vi "ConvertImageToJpg.vi"(11 "buffer":string) -> (1 "image data":T1, 3 "new picture":picture)   [LabVIEW 2017]
uses:
  <vilib>/picture/picture.llb/imagedata.ctl
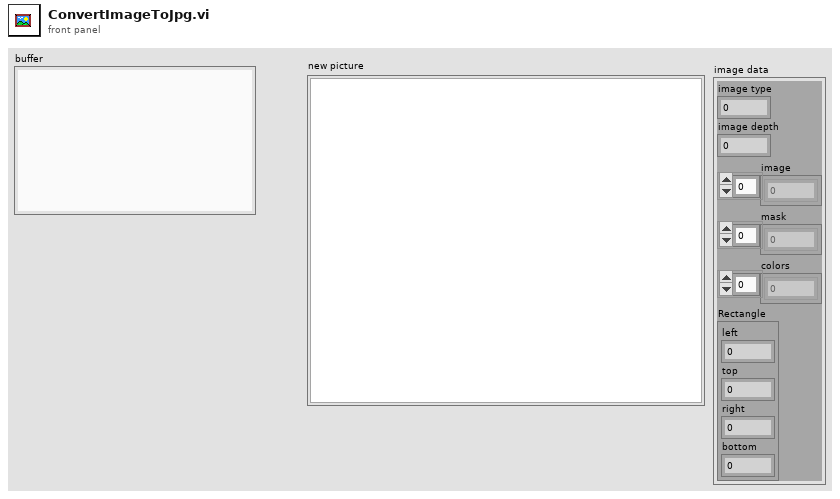
[diagram p1: front panel]
types:
  T1 = typedef "imagedata.ctl" = cluster{"image type":i32, "image depth":i32, "image":u8[], "mask":u8[], "colors":u32[], "Rectangle":cluster{"left":i16, "top":i16, "right":i16, "bottom":i16}}
  T2 = enum16{"big-endian, network order", "native, host order", "little-endian"}
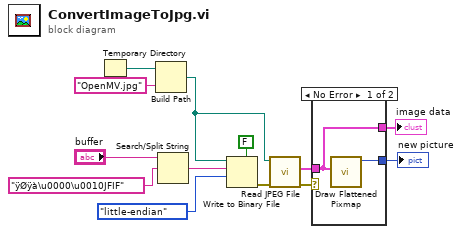
[diagram p0: block diagram]
diagram:
  n1 = Temporary Directory() -> (w4:path)
  n2 = Build Path(base path=w4, name or relative path="OpenMV.jpg") -> (appended path=w2:path)
  n3 = Search/Split String(string="buffer", search string/char (-)="ÿØÿà\u0000\u0010JFIF") -> (match + rest of string=w6:string)  [unwired: 1 in, 2 out]
  n4 = Write to Binary File(file (use dialog)=w2, data=w6, 5:FALSE ("prepend array or string size? (T)"), 9:T2."little-endian" ("byte order (0:big-endian, network order)")) -> (error out=w11:errorcluster)  [unwired: 2 in, 2 out]
  n5 = call <vilib>:"Read JPEG File.vi"("error in (no error)"=w11, "path to JPEG file"=w2) -> ("error out"=w5:errorcluster, "image data"=w10:T1)  [unwired: 7 in, 1 out]
  n6 = case shown="No Error" w5 {
    tunnel: w10 -> [w14 _]
    tunnel: [w15 _] -> w9
    tunnel: [w14 _] -> w1
    frame No Error {
      n7 = call <vilib>:"Draw Flattened Pixmap.vi"("image data"=w14) -> ("new picture"=w15:picture)  [unwired: 8 in]
    }
    frame Error {
    }
  }
  "new picture" <- w9
  "image data" <- w1
